vi "Create.vi"(7 "mode settings":variant, 8 "error in":errorcluster, 9 "number of default channels":i32, 10 "channel settings":variant, 11 "analog input mode in":refnum<class "Analog Input Mode.lvclass">) -> (0 "error out":errorcluster, 1 "channels":refnum<class "Channel.lvclass">[](array[class]), 3 "analog input mode out":refnum<class "Analog Input Mode.lvclass">)   [LabVIEW 2020, in "Scan Engine Scripting.lvlib" / "Analog Input Mode.lvclass"]
uses:
  Analog Input Vrms Mode/Analog Input Mode.lvclass
  Channel Classes/Channel/Channel.lvclass
  Controls/analog channel settings.ctl
  c7467f32-0586-4349-95a7-92635455094b.vi
  Channel Classes/AI Channel/AI Channel.lvclass
  C:/jenkins/workspace/ercat-custom-device_release_20.4/Custom Device Source/Scripting/Modules/Channel Classes/Channel/Channel.lvclass
  Scan Engine Scripting.lvlib
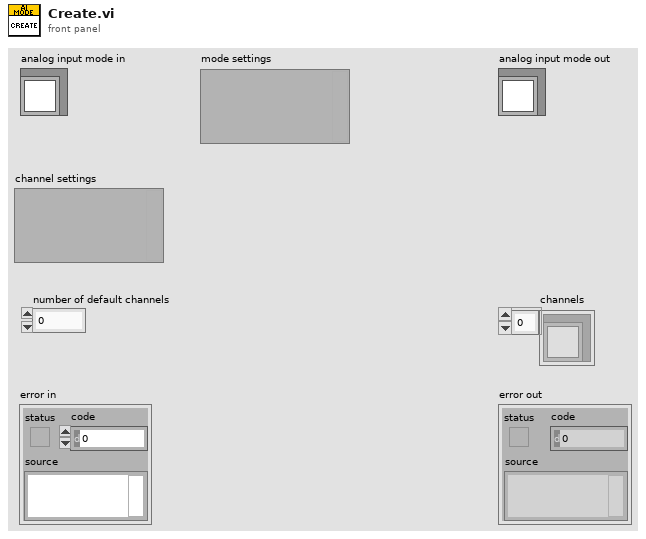
[diagram p1: front panel]
types:
  T1 = typedef "Scan Engine Scripting.lvlib/analog channel settings.ctl" = cluster{"name":string, "default value":dbl}
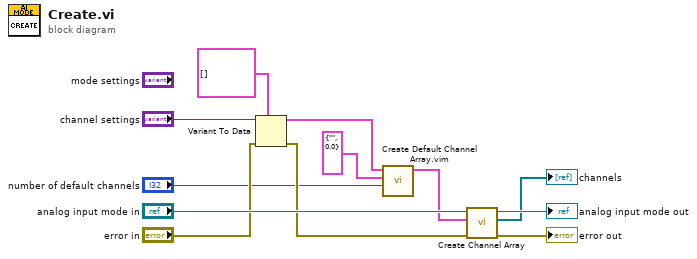
[diagram p0: block diagram]
diagram:
  n1 = Variant To Data(error in="error in", type=T1[] [] ("channel settings"), Variant="channel settings") -> (data=w3:T1[], error out=w6:errorcluster)
  n2 = call "Create Default Channel Array.vim"("number of default channels"="number of default channels", "default settings"=T1 {"name"="", "default value"=0.0} ("channel settings"), "channel settings in"=w3) -> ("channel settings out"=w2:T1[])  [unwired: 8 in]
  n3 = call "Create Channel Array.vi"("error in"=w6, "channel settings"=w2, "analog input mode in"="analog input mode in") -> ("error out"=→"error out":errorcluster, "channels"=→"channels":refnum<class "AI Channel.lvclass">[], "analog input mode out"=→"analog input mode out":refnum<class "Analog Input Mode.lvclass">)  [unwired: 6 in]
